vi "TCP_comms_test.vi"() -> ()   [LabVIEW 2018]
panel:
  out "Sent i":i32
  out "Waveform Chart":i32(graph)
  in  "address":string="127.0.0.1"
  in  "Send many":bool
  in  "Value to send":u32
  in  "Send single value":bool
  out "Received value/i":u32
  out "Connection opened?":bool
  out "Error Out":errorcluster
  in  "Stop and Exit":bool
  in  "Error In":errorcluster
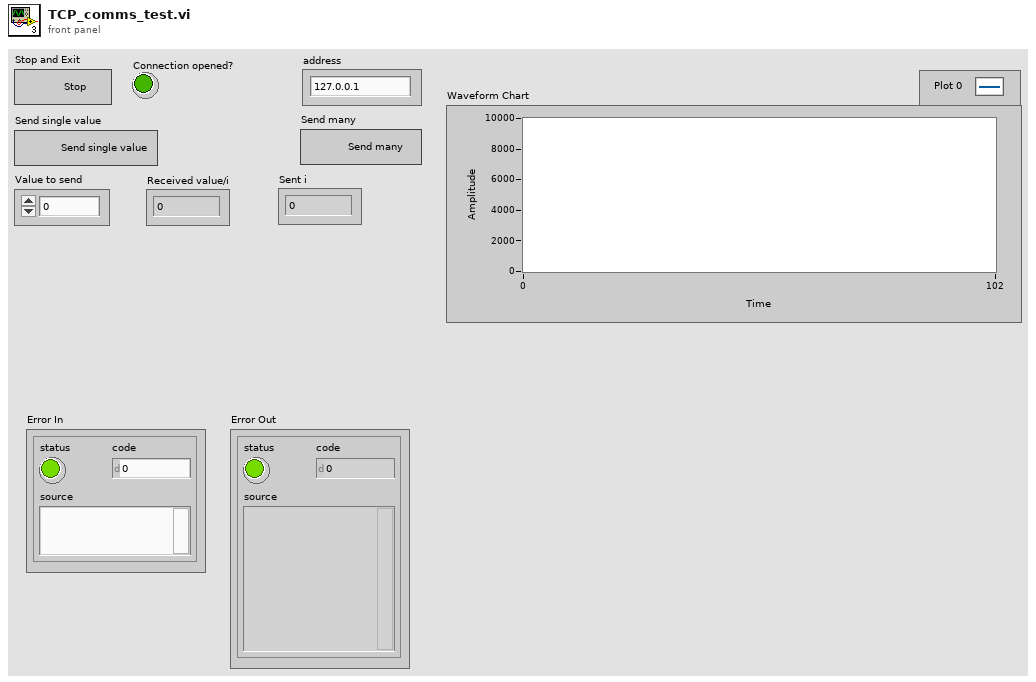
[diagram p1: front panel]
types:
  T1 = enum16{"Standard", "Buffered", "CRLF", "Immediate"}
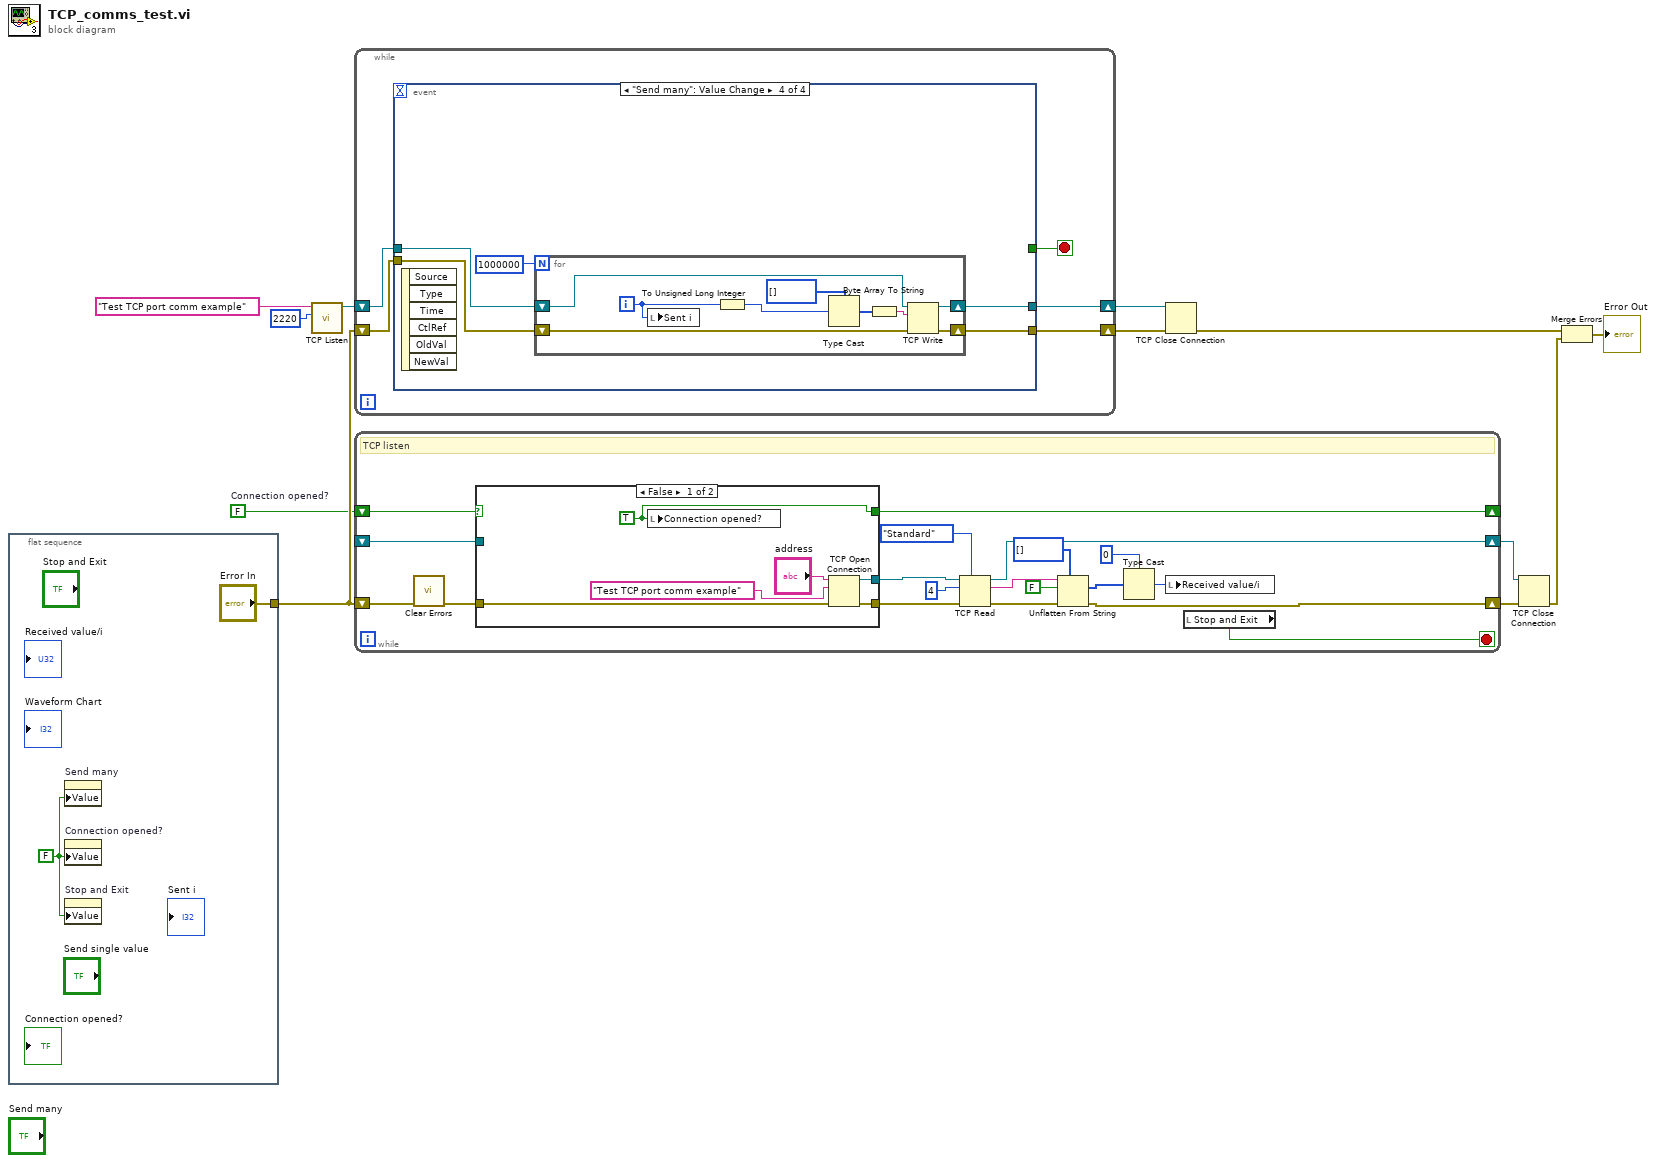
[diagram p0: block diagram]
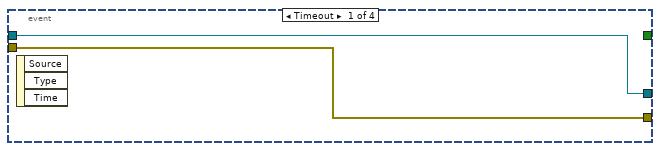
[diagram p3: hidden frame]
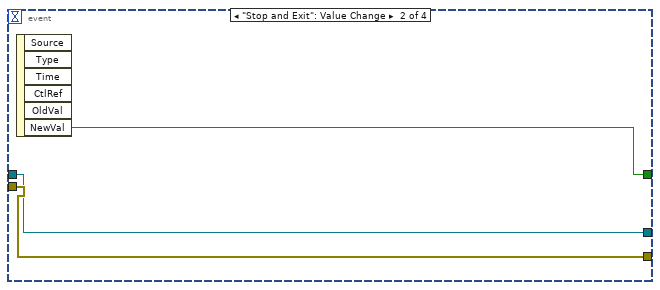
[diagram p4: hidden frame]
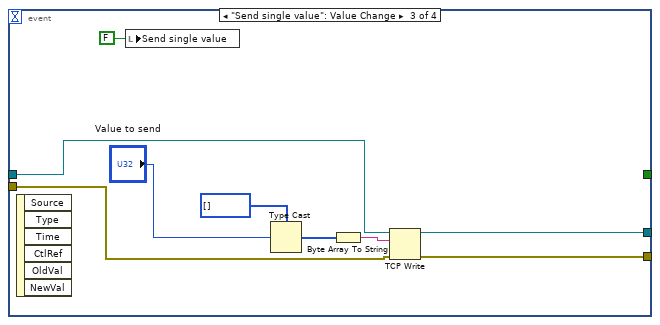
[diagram p5: hidden frame]
diagram:
  w8 = FALSE  # Connection opened?
  n1 = flat-sequence {
    tunnel: ["Error In"] -> w12
    frame #0 {
      w13 = FALSE ("Stop and Exit")
      n2 = property on="Send many" class="Bool (strict)"("Value"=w13) -> ()  [unwired: 2 in, 2 out]
      n3 = property on="Connection opened?" class="Bool (strict)"("Value"=w13) -> ()  [unwired: 2 in, 2 out]
      n4 = property on="Stop and Exit" class="Bool (strict)"("Value"=w13) -> ()  [unwired: 2 in, 2 out]
    }
  }
  n5 = call <vilib>:"TCP Listen.vi"("port"=u16 2220, "service name"="Test TCP port comm example") -> ("connection ID"=w1:refnum<k5>)  [unwired: 5 in, 4 out]
  n6 = while {
    shift-right: [w17] -> w7
    shift-left: w12 -> [w18]
    shift-right: [w15] -> w6
    shift-left: w1 -> [w16]
    stop <- w19 stop-if-true
    n7 = event shown="[3] \"Send many\": Value Change" {
      selector: _ -> [_ _ _ _]
      dyn-events: _ -> [_ _ _ _]
      timeout: _ -> [_ _ _ _]
      tunnel: [_ w24 _ _] -> w19
      tunnel: w18 -> [w21 w23 w31 w36]
      tunnel: [w21 w23 w30 w35] -> w17
      tunnel: w16 -> [w20 w22 w33 w38]
      tunnel: [w20 w22 w32 w37] -> w15
      event Timeout {
        n8 = event-data() -> ()  [unwired: 1 in, 3 out]
      }
      event "Stop and Exit": Value Change {
        n9 = event-data() -> ("NewVal"=w24:bool)  [unwired: 1 in, 5 out]
      }
      event "Send single value": Value Change {
        n10 = event-data() -> ()  [unwired: 1 in, 6 out]
        n11 = local write "Send single value"(FALSE ("Send single value")) -> ()
        n12 = Type Cast(type=u8[] [], x="Value to send") -> (*(type *) &x=w27:u8[])
        n13 = Byte Array To String(unsigned byte array=w27) -> (string=w26:string)
        n14 = TCP Write(connection ID=w33, data in=w26, error in (no error)=w31) -> (connection ID out=w32:refnum<k5>, error out=w30:errorcluster)  [unwired: 1 in, 1 out]
      }
      event "Send many": Value Change {
        n15 = event-data() -> ()  [unwired: 1 in, 6 out]
        n16 = for {
          N: 1000000 -> [_]
          shift-right: [w46] -> w37
          shift-left: w38 -> [w47]
          shift-right: [w44] -> w35
          shift-left: w36 -> [w45]
          i -> [w39]
          n17 = local write "Sent i"(w39) -> ()
          n18 = To Unsigned Long Integer(number=w39) -> (unsigned 32bit integer=w40:u32)
          n19 = Type Cast(type=u8[] [], x=w40) -> (*(type *) &x=w42:u8[])
          n20 = Byte Array To String(unsigned byte array=w42) -> (string=w41:string)
          n21 = TCP Write(connection ID=w47, data in=w41, error in (no error)=w45) -> (connection ID out=w46:refnum<k5>, error out=w44:errorcluster)  [unwired: 1 in, 1 out]
        }
      }
    }
  }
  n22 = while {
    shift-right: [w49] -> w10
    shift-left: w12 -> [w51]
    shift-right: [w64] -> _
    shift-left: w8 -> [w65]
    shift-right: [w60] -> w5
    shift-left: _ -> [w63]
    stop <- w66 stop-if-true
    # "TCP listen"
    n23 = call <vilib>:"Clear Errors.vi"("error in (no error)"=w51) -> ("error out"=w48:errorcluster)  [unwired: 5 in, 1 out]
    n24 = case shown="False" w65 {
      selector: w65 -> [_ w74]
      tunnel: w48 -> [w72 w75]
      tunnel: [w71 w75] -> w62
      tunnel: [w67 w74] -> w64
      tunnel: [w70 w73] -> w61
      tunnel: w63 -> [_ w73]
      frame False {
        w67 = TRUE
        n25 = local write "Connection opened?"(w67) -> ()
        n26 = TCP Open Connection(address="address", remote port or service name="Test TCP port comm example" ("service name"), error in (no error)=w72) -> (connection ID=w70:refnum<k5>, error out=w71:errorcluster)  [unwired: 2 in]
      }
      frame True {
      }
    }
    n27 = TCP Read(connection ID=w61, bytes to read=4, error in (no error)=w62, 7:T1."Standard" ("mode (standard)")) -> (connection ID out=w60:refnum<k5>, data out=w59:string, error out=w58:errorcluster)  [unwired: 1 in]
    n28 = Unflatten From String(type=u8[] [], binary string=w59, data includes array or string size? (T)=FALSE, error in (no error)=w58) -> (value=w54:u8[], error out=w49:errorcluster)  [unwired: 1 in, 1 out]
    n29 = Type Cast(type=0, x=w54) -> (*(type *) &x=w55:i32)
    n30 = local write "Received value/i"(w55) -> ()
    n31 = local read "Stop and Exit"() -> (w66:bool)
  }
  n32 = TCP Close Connection(connection ID=w6, error in (no error)=w7) -> (error out=w4:errorcluster)  [unwired: 1 in, 1 out]
  n33 = TCP Close Connection(connection ID=w5, error in (no error)=w10) -> (error out=w9:errorcluster)  [unwired: 1 in, 1 out]
  n34 = Merge Errors(w4, w9) -> (→"Error Out":errorcluster)
